vi "Color Picker_Main.vi"(7 "error in (no error)":errorcluster, 8 "Window Origin (0,0) In":cluster{"Left":i16, "Top":i16}={"Left"=200, "Top"=200}, 10 "Color In":u32(colorbox)) -> (0 "error out":errorcluster, 1 "Cancled":bool, 3 "Current Color":u32(colorbox))   [LabVIEW 2009]
doc: "Main Program to choose a legal icon color"
uses:
  Controls/Bool_Otagon Stop Button no latch.ctl
  Color Picker Controls/Color Picker_ENUM Commands.ctl
  Color Picker Controls/Color Picker_Array Icon Color Set.ctl
  Color Picker Controls/Color Picker_Cluster Command Data Set.ctl
  Color Picker Controls/Color Picker_ENUM Color Component Select.ctl
panel:
  in  "Cancel Button":bool
  out "Previous Colors":u32[](array[colorbox])
  out "HSL Values":cluster{"Lum:":u8, "Sat:":u8, "Hue:":u8}
  out "RGB Values":cluster{"Blue:":u8, "Green: ":u8, "Red:":u8}
  out "Color Pallet":T1
  out "Current\nCmd":T2=enum."Initialize"
  in  "STOP Program":T3
  # "History"
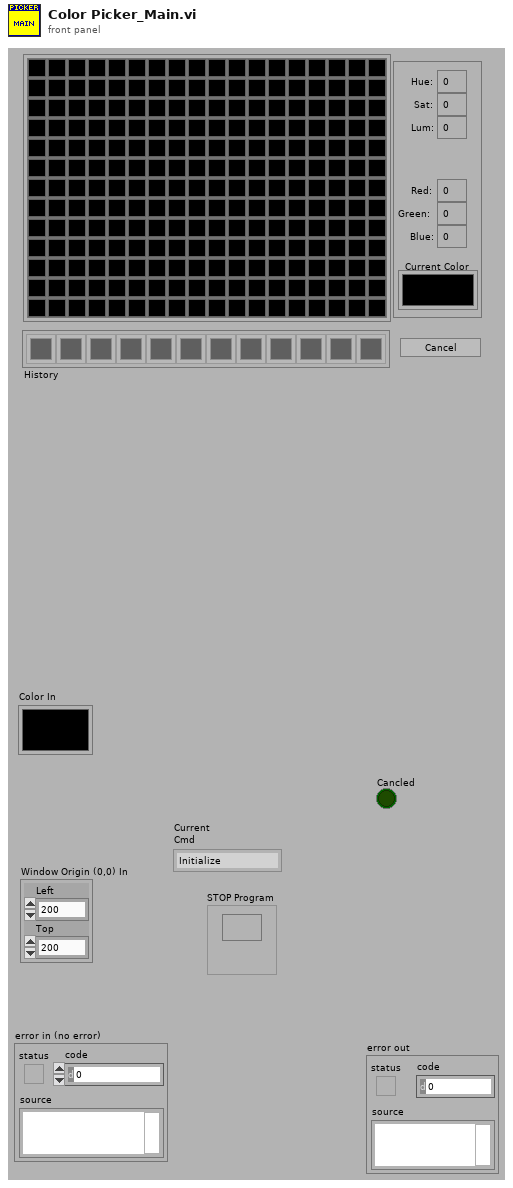
[diagram p1: front panel]
types:
  T1 = typedef "Color Picker_Array Icon Color Set.ctl" = u32[][]
  T2 = typedef "Color Picker_ENUM Commands.ctl" = enum16{"No Command", "Initialize", "Display Color", "Set Position", "Enable FP", "Hide FP", "Stop Program", "Set Original Color"}
  T3 = typedef "Bool_Otagon Stop Button no latch.ctl" = bool
  T4 = typedef "Color Picker_Cluster Command Data Set.ctl" = cluster{"Cmd":T2, "Data":variant}
  T5 = typedef "Color Picker_ENUM Color Component Select.ctl" = enum16{"RGB", "HSL"}
  T6 = enum32{"Invalid", "Standard", "Closed", "Hidden", "Minimized", "Maximized"}
  T7 = typedef "Color Picker_Cluster Color Component Data Set.ctl" = cluster{"Blue (or Light or Val) value":u8, "Green (or Sat) value":u8, "Red (or Hue) value":u8}
  T8 = typedef "LVPoint32TypeDef.ctl" = cluster{"Horizontal":i32, "Vertical":i32}
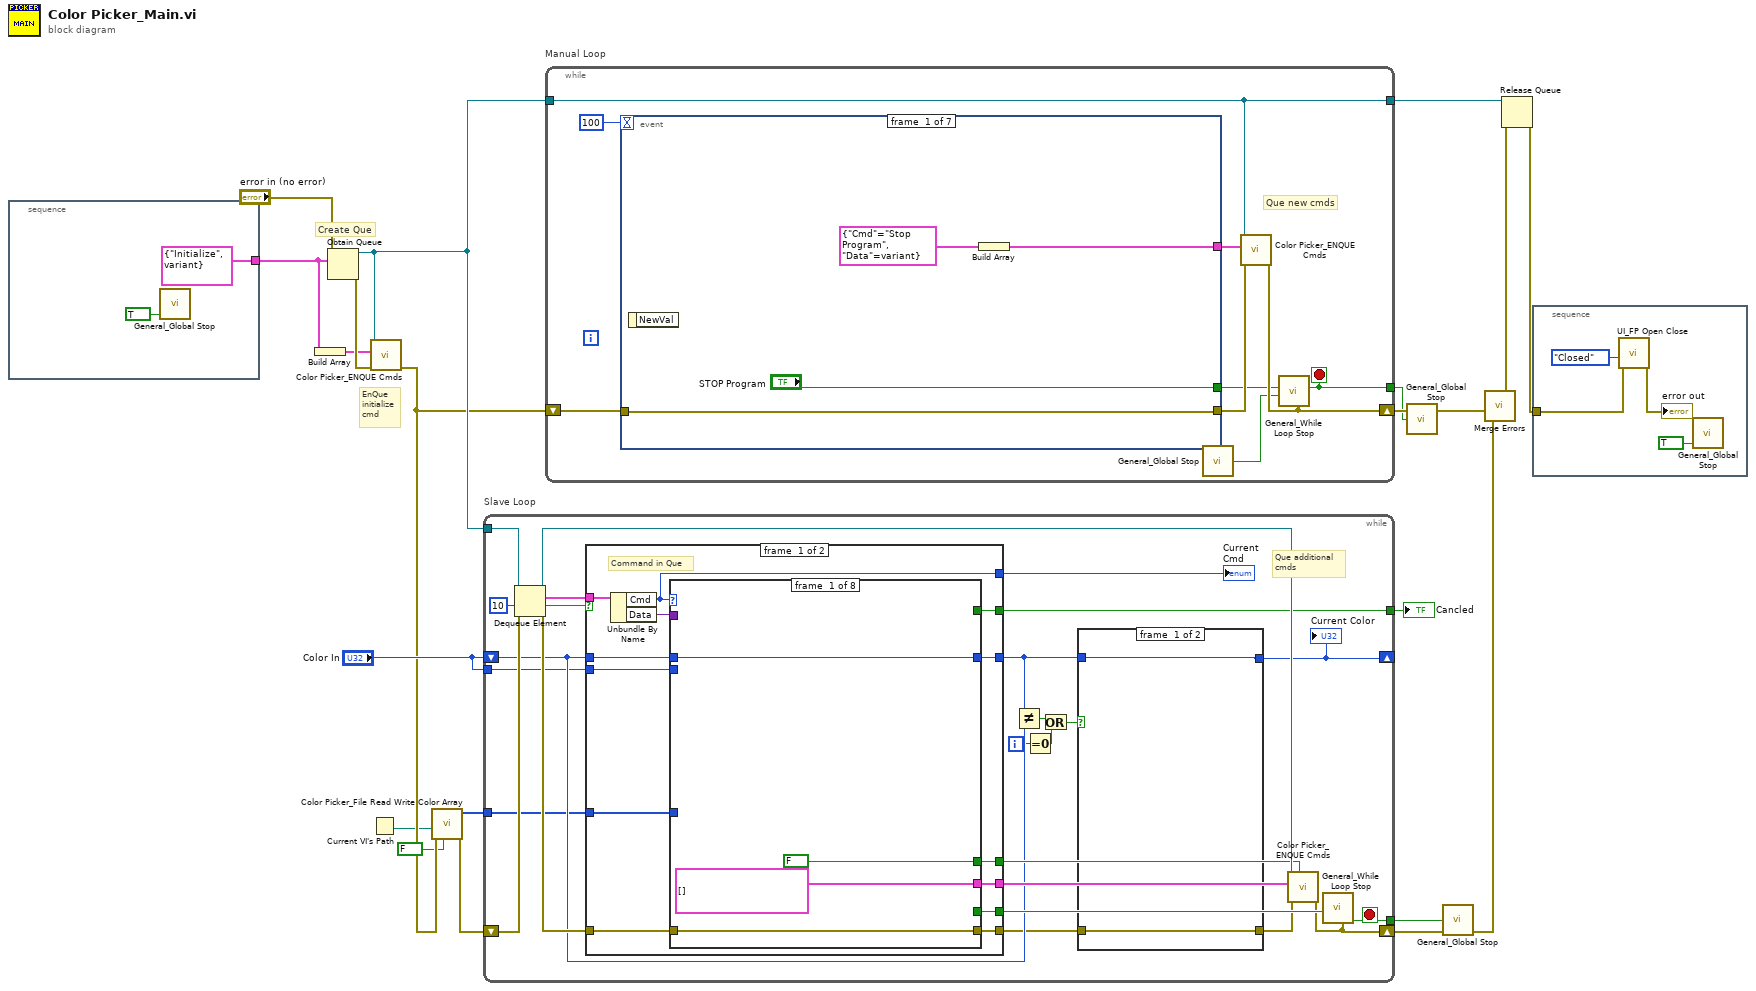
[diagram p0: block diagram]
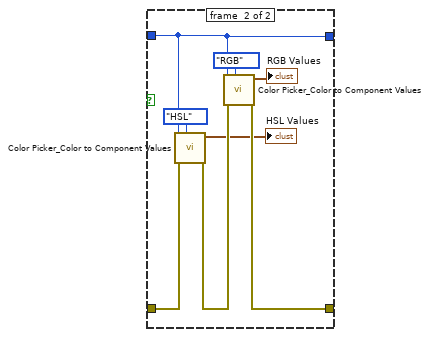
[diagram p2: hidden frame]
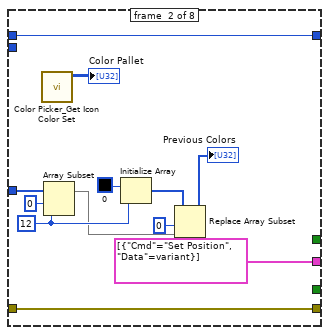
[diagram p3: hidden frame]
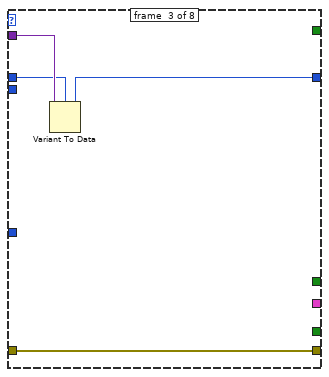
[diagram p4: hidden frame]
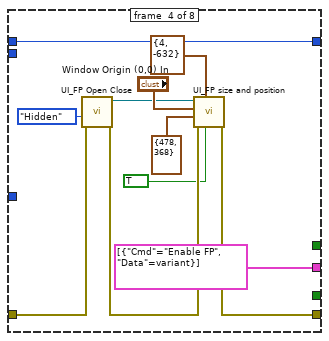
[diagram p5: hidden frame]
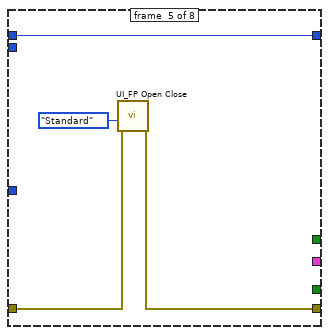
[diagram p6: hidden frame]
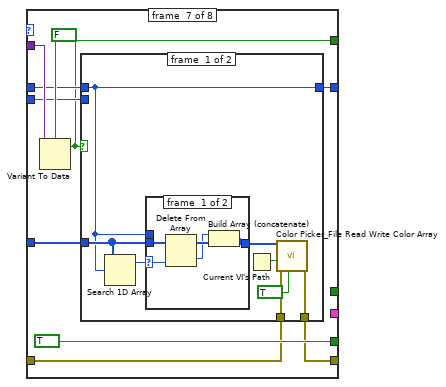
[diagram p8: hidden frame]
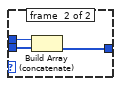
[diagram p9: hidden frame]
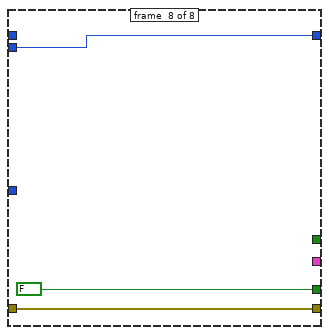
[diagram p11: hidden frame]
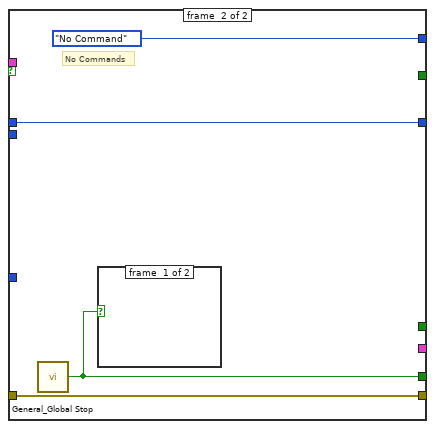
[diagram p12: hidden frame]
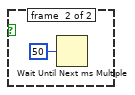
[diagram p13: hidden frame]
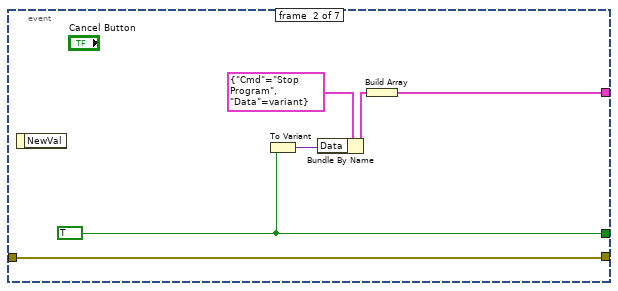
[diagram p14: hidden frame]
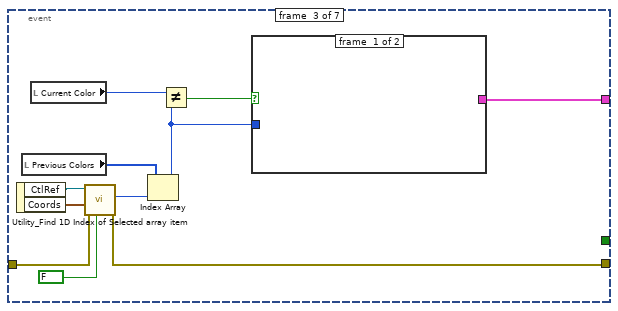
[diagram p15: hidden frame]
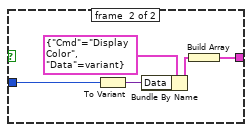
[diagram p16: hidden frame]
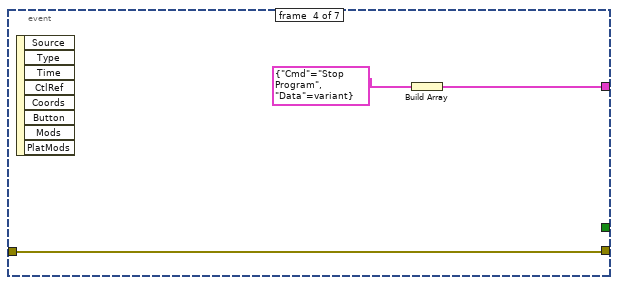
[diagram p17: hidden frame]
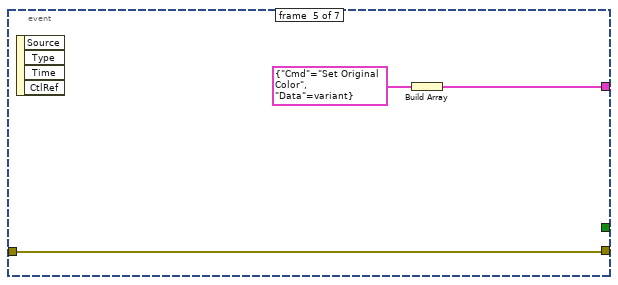
[diagram p18: hidden frame]
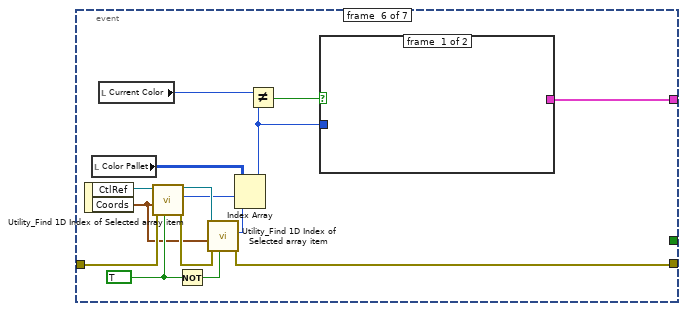
[diagram p19: hidden frame]
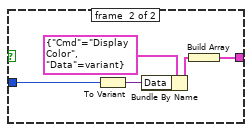
[diagram p20: hidden frame]
diagram:
  # "EnQue\ninitialize\ncmd"
  # "Create Que"
  n1 = stacked-sequence {
    tunnel: [T4 {"Cmd"=enum."Initialize", "Data"=variant} ("Cluster")] -> w12
    frame #0 {
      n2 = call "General_Global Stop.vi"("Complete"=TRUE ("reset")) -> ()  [unwired: 4 in, 1 out]
    }
  }
  n3 = Build Array(w12) -> (w11:T4[])
  n4 = Obtain Queue(element data type=w12, error in (no error)="error in (no error)") -> (queue out=w13:refnum<queue>, error out=w14:errorcluster)  [unwired: 3 in, 1 out]
  n5 = Current VI's Path() -> (path=w1:path)
  n6 = call "Color Picker_ENQUE Cmds.vi"("Error"=w14, "Array"=w11, "Queue"=w13) -> ("Error Out"=w4:errorcluster)  [unwired: 8 in]
  n7 = call "Color Picker_File Read Write Color Array.vi"("Read(f)\nWrite(t)"=FALSE ("Read(f)\nWrite(t)"), "Error"=w4, "Home Path"=w1) -> ("Error Out"=w3:errorcluster, "Template Select Out"=w5:u32[])  [unwired: 6 in, 1 out]
  n8 = while "Slave Loop" {
    tunnel: w13 -> [w46]
    shift-right: [w39] -> w16
    shift-left: w3 -> [w44]
    tunnel: [w40] -> w10
    shift-right: [w29] -> _
    shift-left: "Color In" -> [w33]
    tunnel: "Color In" -> [w23]
    tunnel: [w22] -> w6
    tunnel: w5 -> [w24]
    i -> [w27]
    stop <- w40 stop-if-true
    # "Que additional\ncmds"
    n9 = Dequeue Element(queue=w46, timeout in ms (-1)=10, error in (no error)=w44) -> (queue out=w37:refnum<queue>, element=w42:T4, timed out?=w38:bool, error out=w43:errorcluster)
    n10 = case shown="False" w38 {
      tunnel: w43 -> [w69 w141]
      tunnel: w42 -> [w68 _]
      tunnel: [w66 w139] -> w41
      tunnel: [w65 w141] -> w31
      tunnel: [w64 _] -> w36
      tunnel: [w63 _] -> w35
      tunnel: [w62 Color_Picker_ENUM_Commands."No Command" ("Cmd")] -> w34
      tunnel: w33 -> [w61 w138]
      tunnel: [w60 w138] -> w32
      tunnel: w24 -> [w59 _]
      tunnel: w23 -> [w58 _]
      tunnel: [w57 _] -> w22
      frame #0 {
        # "Command in Que"
        n11 = Unbundle By Name(w68) -> ("Cmd"=w62:T2, "Data"=w67:variant)
        n12 = case shown="\"Set Position\"" w62 {
          tunnel: w69 -> [w73 w85 w89 w97 w103 w106 w108 w135]
          tunnel: [w73 w85 w89 w91 w102 w106 w107 w135] -> w65
          tunnel: w67 -> [_ _ w88 _ _ _ w115 _]
          tunnel: [_ _ _ _ _ _ TRUE FALSE] -> w66
          tunnel: [T4[] [] ("appended array") T4[] [{"Cmd"=enum."Set Position", "Data"=variant}] ("appended array") _ T4[] [{"Cmd"=enum."Enable FP", "Data"=variant}] ("appended array") _ _ _ _] -> w64
          tunnel: [FALSE _ _ _ _ _ _ _] -> w63
          tunnel: [w72 w84 w86 w100 w104 w105 w110 w136] -> w60
          tunnel: w61 -> [w72 w84 w87 w100 w104 w105 w112 _]
          tunnel: w59 -> [_ w80 _ _ _ _ w113 _]
          tunnel: w58 -> [_ _ _ _ _ _ w111 w136]
          tunnel: [_ _ _ _ _ _ w109 _] -> w57
          frame #0 {
          }
          frame #1 {
            w79 = 12 ("length")
            n13 = call "Color Picker_Get Icon Color Set.vi"() -> ("Icon Color Set Out"=→"Color Pallet":T1)  [unwired: 9 in, 2 out]
            n14 = Array Subset(array=w80, index=0, length=w79) -> (w76:u32[])
            n15 = Initialize Array(u32 0 ("Color Box"), w79) -> (w77:u32[])
            n16 = Replace Array Subset(array=w77, new element=w76, index=0) -> (→"Previous Colors":u32[])
          }
          frame #2 {
            n17 = Variant To Data(Variant=w88, type=w87) -> (data=w86:u32)  [unwired: 1 in, 1 out]
          }
          frame #3 {
            n18 = call "UI_FP Open Close.vi"("Error"=w97, "State"=T6."Hidden") -> ("Error Out"=w92:errorcluster, "Dup Ref Out"=w93:refnum<vi>)  [unwired: 8 in]
            n19 = call "UI_FP size and position.vi"("Move Window (f) In"=TRUE, "FP Origin (0,0) In"=cluster{"Horizontal":i16, "Vertical":i16} {"Horizontal"=4, "Vertical"=-632}, "Error In"=w92, "Window Size(No Resize) In"=cluster{"Width":i16, "Height":i16} {"Width"=478, "Height"=368}, "Window Origin (0,0) In"="Window Origin (0,0) In", "Vi Ref (this Vi) In"=w93) -> ("Error Out"=w91:errorcluster)  [unwired: 4 in, 1 out]
          }
          frame #4 {
            n20 = call "UI_FP Open Close.vi"("Error"=w103, "State"=T6."Standard") -> ("Error Out"=w102:errorcluster)  [unwired: 8 in, 1 out]
          }
          frame #5 {
          }
          frame #6 {
            n21 = Variant To Data(Variant=w115, type=FALSE) -> (data=w109:bool)  [unwired: 1 in, 1 out]
            n22 = case shown="False" w109 {
              tunnel: w113 -> [w123 _]
              tunnel: w112 -> [w122 _]
              tunnel: w111 -> [_ w134]
              tunnel: [w122 w134] -> w110
              tunnel: w108 -> [w120 w133]
              tunnel: [w119 w133] -> w107
              frame #0 {
                n23 = Search 1D Array(1D array=w123, element=w122) -> (index of element=w124:i32)  [unwired: 1 in]
                n24 = case shown="Default" w124 {
                  selector: w124 -> [w128 _]
                  tunnel: [w125 w132] -> w121
                  tunnel: w123 -> [w129 w131]
                  tunnel: w122 -> [_ w130]
                  frame #0 {
                    n25 = Delete From Array(array=w129, index=w128) -> (deleted portion=w126:u32, array with subset deleted=w127:u32[])  [unwired: 1 in]
                    n26 = Build Array (concatenate)(w126, w127) -> (w125:u32[])
                  }
                  frame #1 {
                    n27 = Build Array (concatenate)(w130, w131) -> (w132:u32[])
                  }
                }
                n28 = Current VI's Path() -> (path=w117:path)
                n29 = call "Color Picker_File Read Write Color Array.vi"("Read(f)\nWrite(t)"=TRUE ("Read(f)\nWrite(t)"), "Error"=w120, "Home Path"=w117, "Template Select"=w121) -> ("Error Out"=w119:errorcluster)  [unwired: 5 in, 2 out]
              }
              frame #1 {
              }
            }
          }
          frame #7 {
          }
        }
      }
      frame #1 {
        # "No Commands"
        n30 = call "General_Global Stop.vi"() -> ("Output"=w139:T3)  [unwired: 5 in]
        n31 = case shown="True" w139 {
          frame #0 {
          }
          frame #1 {
            n32 = Wait Until Next ms Multiple(millisecond multiple=u32 50) -> ()  [unwired: 1 out]
          }
        }
      }
    }
    "Current\nCmd" <- w34
    n33 = Not Equal?(x=w32, y=w33) -> (x != y?=w28:bool)
    n34 = Equal To 0?(x=w27) -> (x = 0?=w25:bool)
    n35 = Or(x=w28, y=w25) -> (x .or. y?=w26:bool)
    n36 = case shown="True" w26 {
      tunnel: w32 -> [w48 w49]
      tunnel: w31 -> [w47 w54]
      tunnel: [w47 w52] -> w30
      tunnel: [w48 w49] -> w29
      frame #0 {
      }
      frame #1 {
        n37 = call "Color Picker_Color to Component Values.vi"("Select Conversion"=Color_Picker_ENUM_Color_Component_Select."HSL", "Error"=w54, "Color"=w49) -> ("Error Out"=w53:errorcluster, "Color Value Out"=→"HSL Values":T7)  [unwired: 7 in]
        n38 = call "Color Picker_Color to Component Values.vi"("Select Conversion"=Color_Picker_ENUM_Color_Component_Select."RGB", "Error"=w53, "Color"=w49) -> ("Error Out"=w52:errorcluster, "Color Value Out"=→"RGB Values":T7)  [unwired: 7 in]
      }
    }
    "Current Color" <- w29
    n39 = call "Color Picker_ENQUE Cmds.vi"("Add To Begining"=w35, "Error"=w30, "Array"=w36, "Queue"=w37) -> ("Error Out"=w39:errorcluster)  [unwired: 7 in]
    n40 = call "General_While Loop Stop.vi"("Error In"=w39, "Stop 3 In"=w41) -> ("Stop Out3"=w40:bool)  [unwired: 5 in, 3 out]
  }
  "Cancled" <- w6
  n41 = while "Manual Loop" {
    shift-right: [w147] -> w18
    shift-left: w4 -> [w151]
    tunnel: w13 -> [w144]
    tunnel: [w144] -> w19
    tunnel: [w145] -> w9
    stop <- w145 stop-if-true
    # "Que new cmds"
    n42 = event shown="[3] \"Previous Colors\", \"Color Pallet\", \"Current Color\": Mouse Up" {
      selector: _ -> [_ _ _ _ _ _ _]
      dyn-events: _ -> [_ _ _ _ _ _ _]
      timeout: 100 -> [_ _ _ _ _ _ _]
      tunnel: w151 -> [w154 w161 w167 w178 w181 w197 w205]
      tunnel: [w154 w161 w172 w178 w181 w193 w205] -> w149
      tunnel: ["STOP Program" w157 _ _ _ _ _] -> w146
      tunnel: [w153 w160 w171 w179 w182 w198 _] -> w148
      event #0 {
        n43 = event-data() -> ()  [unwired: 1 in, 1 out]
        n44 = Build Array(T4 {"Cmd"=enum."Stop Program", "Data"=variant} ("element")) -> (w153:T4[])
      }
      event #1 {
        w157 = T3 TRUE ("STOP Program")
        n45 = event-data() -> ()  [unwired: 1 in, 1 out]
        n46 = To Variant(anything=w157) -> (Variant=w156:variant)
        n47 = Bundle By Name(cluster=T4 {"Cmd"=enum."Stop Program", "Data"=variant} ("element"), "Data"=w156) -> (w158:T4)
        n48 = Build Array(w158) -> (w160:T4[])
      }
      event #2 {
        n49 = event-data() -> ("CtlRef"=w169:refnum<vi>, "Coords"=w168:T8)  [unwired: 1 in]
        n50 = local read "Previous Colors"() -> (w165:u32[])
        n51 = local read "Current Color"() -> (w163:u32)
        n52 = call "Utility_Find 1D Index of Selected array item.vi"("Vertical(t)\nHorizontal(f)"=FALSE ("Vertical(t)\nHorizontal(f)"), "Error"=w167, "Mouse Cord"=w168, "Array REf"=w169) -> ("Error Out"=w172:errorcluster, "Index Out"=w170:i32)  [unwired: 4 in, 2 out]
        n53 = Index Array(array=w165, index=w170) -> (element=w164:u32)
        n54 = Not Equal?(x=w163, y=w164) -> (x != y?=w162:bool)
        n55 = case shown="True" w162 {
          tunnel: [_ w177] -> w171
          tunnel: w164 -> [_ w173]
          frame #0 {
          }
          frame #1 {
            n56 = To Variant(anything=w173) -> (Variant=w175:variant)
            n57 = Bundle By Name(cluster=T4 {"Cmd"=enum."Display Color", "Data"=variant} ("element"), "Data"=w175) -> (w174:T4)
            n58 = Build Array(w174) -> (w177:T4[])
          }
        }
      }
      event #3 {
        n59 = event-data() -> ()  [unwired: 1 in, 8 out]
        n60 = Build Array(T4 {"Cmd"=enum."Stop Program", "Data"=variant} ("element")) -> (w179:T4[])
      }
      event #4 {
        n61 = event-data() -> ()  [unwired: 1 in, 4 out]
        n62 = Build Array(T4 {"Cmd"=enum."Set Original Color", "Data"=variant} ("element")) -> (w182:T4[])
      }
      event #5 {
        w192 = TRUE ("Vertical(t)\nHorizontal(f)")
        n63 = event-data() -> ("CtlRef"=w189:refnum<vi>, "Coords"=w190:T8)  [unwired: 1 in]
        n64 = local read "Color Pallet"() -> (w185:T1)
        n65 = local read "Current Color"() -> (w196:u32)
        n66 = call "Utility_Find 1D Index of Selected array item.vi"("Vertical(t)\nHorizontal(f)"=w192, "Error"=w197, "Mouse Cord"=w190, "Array REf"=w189) -> ("Error Out"=w194:errorcluster, "Index Out"=w186:i32, "Array REf Out"=w188:refnum<vi>)  [unwired: 4 in, 1 out]
        n67 = Not(x=w192) -> (.not. x?=w191:bool)
        n68 = call "Utility_Find 1D Index of Selected array item.vi"("Vertical(t)\nHorizontal(f)"=w191, "Error"=w194, "Mouse Cord"=w190, "Array REf"=w188) -> ("Error Out"=w193:errorcluster, "Index Out"=w187:i32)  [unwired: 4 in, 2 out]
        n69 = Index Array(array=w185, index (row)=w186, index (col)=w187) -> (element=w184:u32)
        n70 = Not Equal?(x=w196, y=w184) -> (x != y?=w195:bool)
        n71 = case shown="True" w195 {
          tunnel: [_ w203] -> w198
          tunnel: w184 -> [_ w199]
          frame #0 {
          }
          frame #1 {
            n72 = To Variant(anything=w199) -> (Variant=w201:variant)
            n73 = Bundle By Name(cluster=T4 {"Cmd"=enum."Display Color", "Data"=variant} ("element"), "Data"=w201) -> (w200:T4)
            n74 = Build Array(w200) -> (w203:T4[])
          }
        }
      }
      event #6 {
        n75 = event-data() -> ()  [unwired: 1 in, 3 out]
        n76 = property class="VI"("Front Panel.IsFrontmost"=TRUE ("Front Panel Window:Is Frontmost")) -> ()  [unwired: 2 in, 2 out]
      }
    }
    n77 = call "General_Global Stop.vi"() -> ("Output"=w143:T3)  [unwired: 5 in]
    n78 = call "Color Picker_ENQUE Cmds.vi"("Error"=w149, "Array"=w148, "Queue"=w144) -> ("Error Out"=w147:errorcluster)  [unwired: 8 in]
    n79 = call "General_While Loop Stop.vi"("Error In"=w147, "Stop 3 In"=w143, "Stop 2 In"=w146) -> ("Stop Out2"=w145:bool)  [unwired: 4 in, 3 out]
  }
  n80 = call "General_Global Stop.vi"("Set"=w9) -> ()  [unwired: 4 in, 1 out]
  n81 = call "General_Global Stop.vi"("Set"=w10) -> ()  [unwired: 4 in, 1 out]
  n82 = call <vilib>:"Merge Errors.vi"("error in 3 (no error)"=w18, "error in 2 (no error)"=w16) -> ("error out"=w17:errorcluster)  [unwired: 5 in]
  n83 = Release Queue(queue=w19, error in (no error)=w17) -> (error out=w15:errorcluster)  [unwired: 1 in, 2 out]
  n84 = stacked-sequence {
    tunnel: w15 -> [w207]
    frame #0 {
      n85 = call "UI_FP Open Close.vi"("Error"=w207, "State"=T6."Closed") -> ("Error Out"=→"error out":errorcluster)  [unwired: 8 in, 1 out]
      n86 = call "General_Global Stop.vi"("Complete"=TRUE ("reset")) -> ()  [unwired: 4 in, 1 out]
    }
  }
